vi "Port Reverse.vi"(3 "error in":errorcluster, 4 "local TCP port":i32=-1, 5 "remote TCP port":i32=-1, 6 "adb location":string) -> (0 "error out":errorcluster, 1 "standard error":string, 2 "standard output":string)   [LabVIEW 2016]
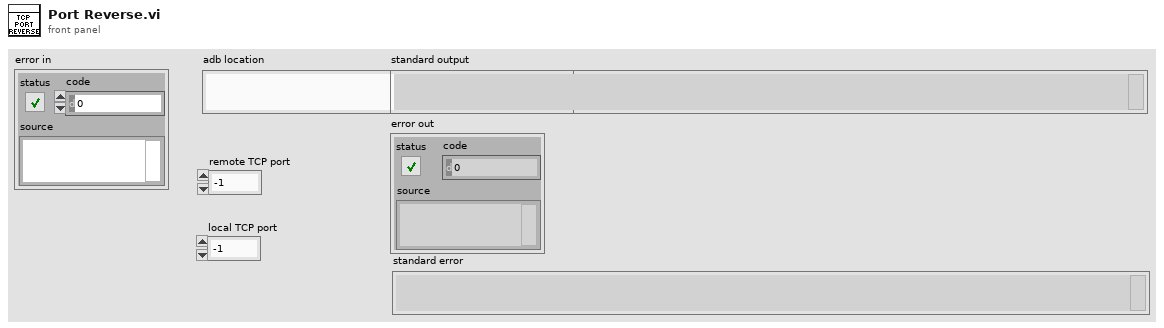
[diagram p1: front panel]
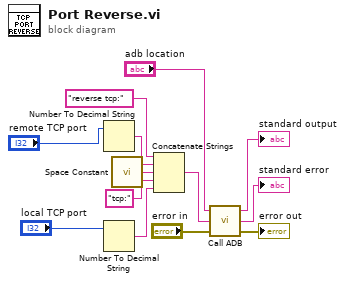
[diagram p0: block diagram]
diagram:
  n1 = Number To Decimal String(number="remote TCP port") -> (decimal integer string=w10:string)  [unwired: 1 in]
  n2 = Number To Decimal String(number="local TCP port") -> (decimal integer string=w6:string)  [unwired: 1 in]
  n3 = call <vilib>:"Space Constant.vi"() -> ("String"=w9:string)
  n4 = Concatenate Strings("reverse tcp:", w10, w9, "tcp:" ("string"), w6) -> (w5:string)
  n5 = call "Call ADB.vi"("error in"="error in", "adb sub-command"=w5, "adb location"="adb location") -> ("error out"=→"error out":errorcluster, "standard error"=→"standard error":string, "standard output"=→"standard output":string)
